vi "Update Coefficients.vi"(8 "error in (no error)":errorcluster, 10 "coeffs":dbl[](array[numeric]), 11 "Node Ref":refnum<data-value>) -> (0 "error out":errorcluster)   [LabVIEW 2013, in "Polynomial Scale editor node.lvclass"]
uses:
  Polynomial Scale editor node.lvclass
  <vilib>/NI/Tag Bus Data Framework/Configuration Editor/Classes/Module editor node/module editor node.lvclass
  module/configuration/Polynomial Scale configuration.lvclass
  <vilib>/NI/DCAF Modules/DCAF Scaling/editor node/Scaling editor node.lvclass
  <vilib>/NI/DCAF Modules/DCAF Scaling/editor node/Scaling editor node.lvclass/Scaling editor node.ctl
  <vilib>/NI/DCAF Modules/DCAF Scaling/editor node/accessors/Read active scale index .vi
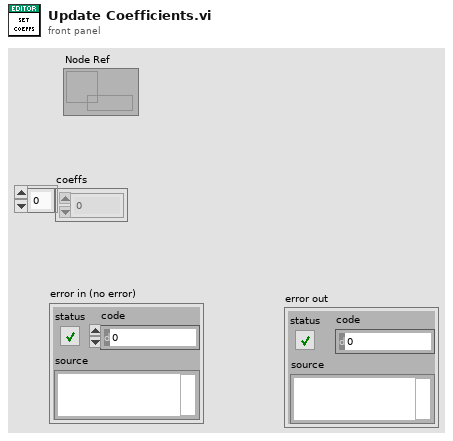
[diagram p1: front panel]
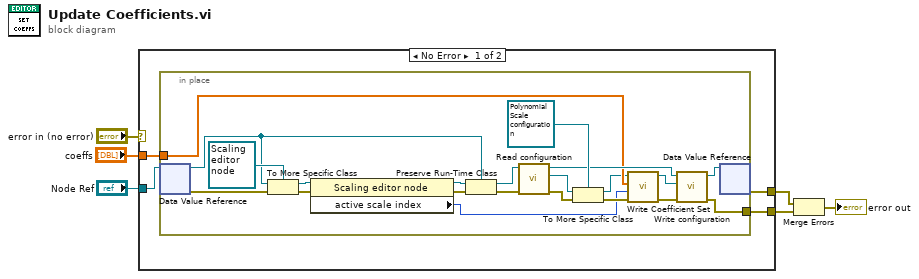
[diagram p0: block diagram]
diagram:
  n1 = case shown="No Error" "error in (no error)" {
    selector: "error in (no error)" -> [_ w32]
    tunnel: "coeffs" -> [w10 _]
    tunnel: [w9 w32] -> w4
    tunnel: [w8 _] -> w3
    tunnel: "Node Ref" -> [w7 _]
    frame No Error {
      n2 = in-place {
        in-place-border: w10 -> [w24]
        in-place-border: [w27] -> w8
        n3 = in-place-dvr #1(w7) -> (w17:refnum<class "module editor node.lvclass">, w19:errorcluster)
        n4 = To More Specific Class(target class=refnum<class "Scaling editor node.lvclass"> refnum ("Scaling editor node"), reference=w17, error in=w19) -> (specific class reference=w21:refnum<class "Scaling editor node.lvclass">, error out=w20:errorcluster)
        n5 = property class="Scaling editor node"(reference=w21, error in=w20) -> (reference out=w18:refnum<class "Scaling editor node.lvclass">, error out=w14:errorcluster, "active scale index "=w13:i32)
        n6 = Preserve Run-Time Class(object in=w18, error in=w14, 2:w17) -> (object out=w11:refnum<class "module editor node.lvclass">, error out=w23:errorcluster)
        n7 = call-dynamic "Read configuration.vi"("error in"=w23, "NISE_CEF_serializable node in"=w11) -> ("error out"=w30:errorcluster, "configuration"=w31:refnum<class "NISE_CEF_serializable configuration.lvclass">, "NISE_CEF_serializable node out"=w28:refnum<class "module editor node.lvclass">)  [unwired: 7 in]
        n8 = To More Specific Class(target class=refnum<class "Polynomial Scale configuration.lvclass"> refnum ("Polynomial Scale configuration"), reference=w31, error in=w30) -> (specific class reference=w16:refnum<class "Polynomial Scale configuration.lvclass">, error out=w15:errorcluster)
        n9 = call "Write Coefficient Set.vi"("error in (no error)"=w15, "scale index"=w13, "Coefficients"=w24, "Polynomial Scale configuration in"=w16) -> ("error out"=w25:errorcluster, "Polynomial Scale configuration out"=w26:refnum<class "Polynomial Scale configuration.lvclass">)  [unwired: 6 in]
        n10 = call-dynamic "Write configuration.vi"("error in"=w25, "configuration"=w26, "NISE_CEF_serializable node in"=w28) -> ("error out"=w27:errorcluster, "NISE_CEF_serializable node out"=w12:refnum<class "module editor node.lvclass">)  [unwired: 7 in]
        n11 = in-place-dvr #1(w12) -> (w9:errorcluster)  [unwired: 1 out]
      }
    }
    frame Error {
    }
  }
  n12 = Merge Errors(w4, w3) -> (→"error out":errorcluster)
